vi "Init Base.vi"(6 "instVIref":T1, 9 "target structure name":string, 11 "target in":refnum<class "Base Target.lvclass">) -> (3 "target out":refnum<class "Base Target.lvclass">)   [LabVIEW 2020, in "NI_TargetHelper.lvlib" / "Base Target.lvclass"]
uses:
  <vilib>/TargetSupport/NI_TargetHelper/Base Target/Base Target.lvclass
  <vilib>/TargetSupport/NI_TargetHelper/Instance VIref.ctl
  <vilib>/TargetSupport/NI_TargetHelper/NetCPU/NetCPU.lvclass
  e:/builds/penguin/labview/branches/2020/dev/dist/vi.lib/TargetSupport/NI_TargetHelper/Base Target/Base Target.lvclass
  <vilib>/TargetSupport/NI_TargetHelper/RTTarget/RTTarget.lvclass
  <vilib>/TargetSupport/NI_TargetHelper/FPGATarget/FPGATarget.lvclass
  <vilib>/TargetSupport/NI_TargetHelper/NI_TargetHelper.lvlib
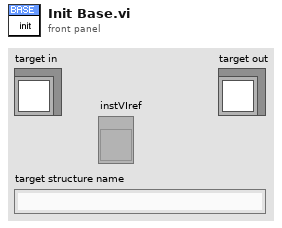
[diagram p1: front panel]
types:
  T1 = typedef "NI_TargetHelper.lvlib/Instance VIref.ctl" = refnum<vi>
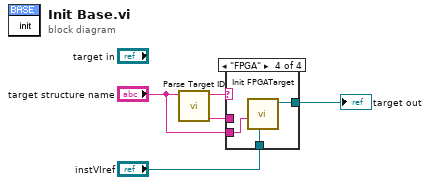
[diagram p0: block diagram]
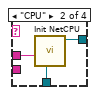
[diagram p3: hidden frame]
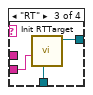
[diagram p4: hidden frame]
diagram:
  n1 = call <vilib>:"Parse Target ID.vi"("targetID"="target structure name") -> ("target location"=w4:string, "target name"=w5:string)  [unwired: 9 in]
  n2 = case shown="\"FPGA\"" w5 {
    tunnel: w4 -> [_ w8 _ _]
    tunnel: [_ w7 w11 w14] -> w1
    tunnel: "instVIref" -> [_ w6 w10 w13]
    tunnel: "target structure name" -> [_ _ w9 w12]
    frame Default {
    }
    frame "CPU" {
      n3 = call <vilib>:"Init NetCPU.vi"("instVIref"=w6, "target location"=w8) -> ("NetCPU out"=w7:refnum<class "NetCPU.lvclass">)  [unwired: 9 in]
    }
    frame "RT" {
      n4 = call <vilib>:"Init RTTarget.vi"("instVIref"=w10, "target structure name"=w9) -> ("RTTarget out"=w11:refnum<class "RTTarget.lvclass">)  [unwired: 9 in]
    }
    frame "FPGA" {
      n5 = call <vilib>:"Init FPGATarget.vi"("instVIref"=w13, "target structure name"=w12) -> ("FPGAtarget out"=w14:refnum<class "FPGATarget.lvclass">)  [unwired: 9 in]
    }
  }
  "target out" <- w1
